vi "Untitled 31.vi"() -> ()   [LabVIEW 2019]
panel:
  out "number":dbl
  out "Moyen":dbl
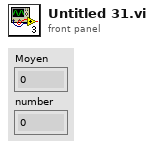
[diagram p1: front panel]
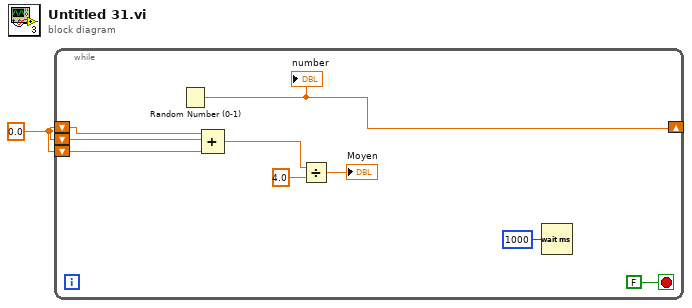
[diagram p0: block diagram]
diagram:
  w1 = 0.0 ("number: 0 to 1")
  n1 = while {
    shift-right: [w10] -> _
    shift-left: w1 -> [w9]
    shift-left: w1 -> [w8]
    shift-left: w1 -> [w7]
    stop <- FALSE stop-if-true
    n2 = Random Number (0-1)() -> (number: 0 to 1=w10:dbl)
    "number" <- w10
    n3 = Compound Arithmetic op=ADD(w9, w8, w7) -> (w6:dbl)
    n4 = Divide(x=w6, y=4.0) -> (x/y=→"Moyen":dbl)
    n5 = Wait (ms)(milliseconds to wait=u32 1000) -> ()  [unwired: 1 out]
  }
